vi "Method Memory.vi"(8 "error in":errorcluster, 11 "Method Name":string) -> (0 "error out":errorcluster, 1 "method exists?":bool, 3 "Method Out":T1)   [LabVIEW 2012]
uses:
  Method.ctl
  ReadWrite.ctl
  Which method type.ctl
panel:
  out "method":i32
  out "version":i32
  out "Version List":i32[](array[numeric])
  in  "Method Failure":T1={"Title"="Method Failure", "About"="5", "Input Parameters"=[], "AutoCAD drawings"=[], "Stock file names"=[], "Publish files"=[], "Display images"=[]}
  out "Method Array (method, version)":T1[][](array[typedef])
  out "Method List":string[](array[string])
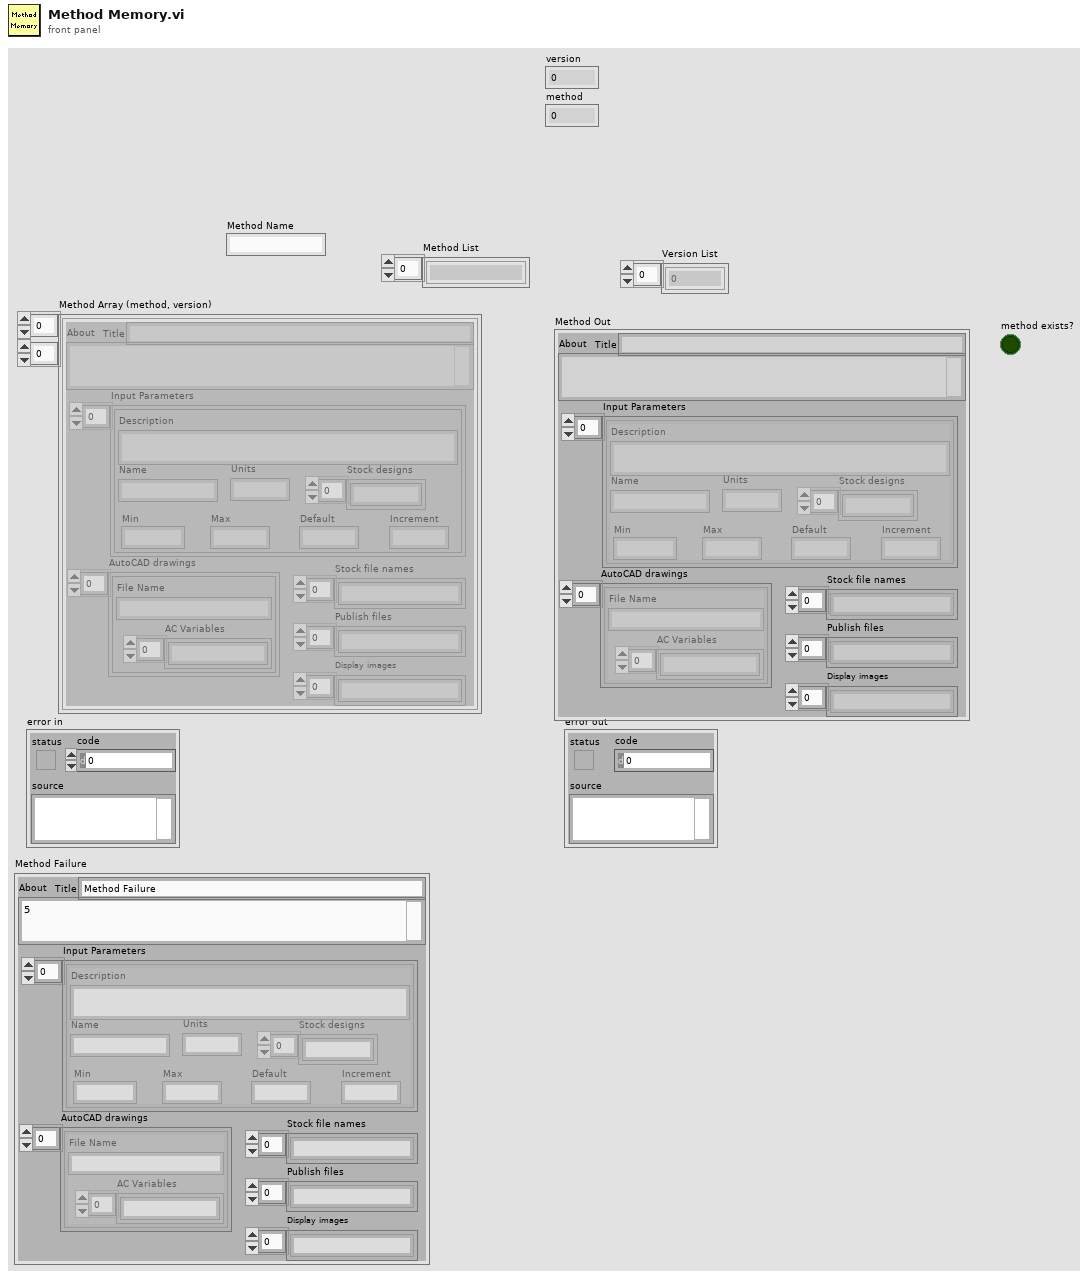
[diagram p1: front panel]
types:
  T1 = typedef "Method.ctl" = cluster{"Title":string, "About":string, "Input Parameters":cluster{"Description":string, "Name":string, "Min":string, "Max":string, "Default":string, "Units":string, "Increment":string, "Stock designs":string[]}[], "AutoCAD drawings":cluster{"File Name":string, "AC Variables":string[]}[], "Stock file names":string[], "Publish files":string[], "Display images":string[]}
  T2 = typedef "ReadWrite.ctl" = enum16{"Read", "Write"}
  T3 = typedef "Which method type.ctl" = enum16{"Master Method", "Method"}
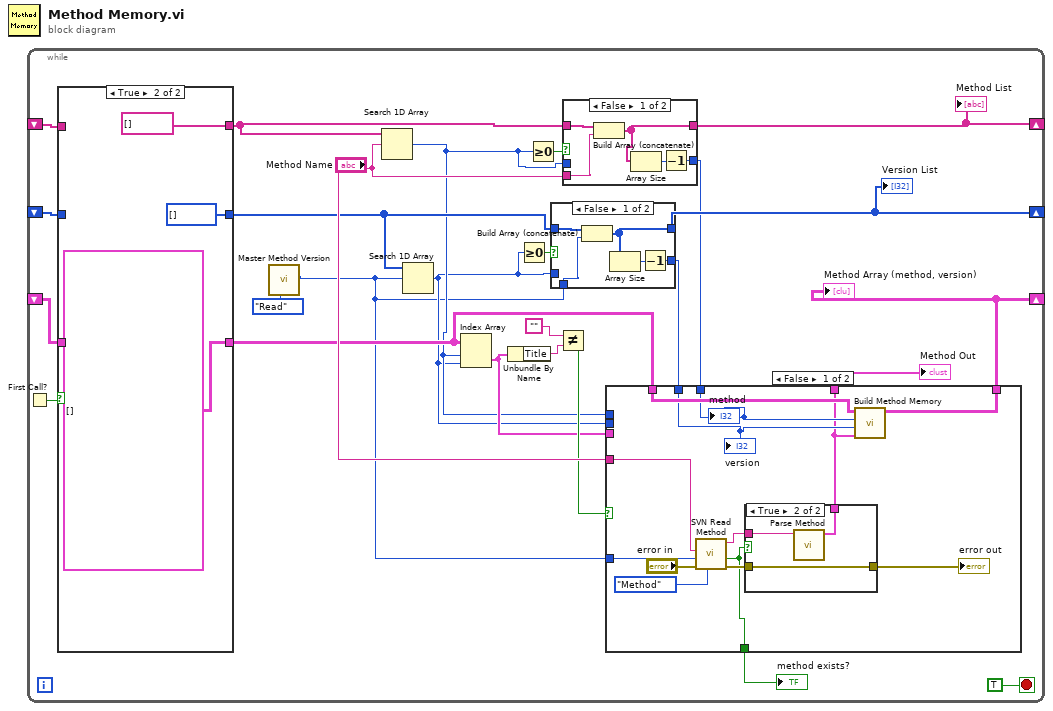
[diagram p0: block diagram]
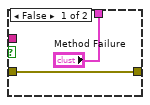
[diagram p4: hidden frame]
diagram:
  n1 = while {
    shift-right: [w23] -> _
    shift-left: _ -> [w16]
    shift-right: [w8] -> _
    shift-left: _ -> [w18]
    shift-right: [w9] -> _
    shift-left: _ -> [w11]
    stop <- TRUE stop-if-true
    n2 = First Call?() -> (First Call?: T/F=w19:bool)
    n3 = case shown="True" w19 {
      tunnel: [w36 T1[][] [] ("Method Array (method, version)")] -> w7
      tunnel: w18 -> [w36 _]
      tunnel: [w35 string[] [] ("Method List")] -> w17
      tunnel: w16 -> [w35 _]
      tunnel: [w34 i32[] []] -> w10
      tunnel: w11 -> [w34 _]
      frame False {
      }
      frame True {
      }
    }
    n4 = call "Master Method Version.vi"("Config"=ReadWrite."Read") -> ("Current Master Method Version"=w1:i32)  [unwired: 7 in, 3 out]
    n5 = Search 1D Array(1D array=w17, element="Method Name") -> (index of element=w4:i32)  [unwired: 1 in]
    n6 = Search 1D Array(1D array=w10, element=w1) -> (index of element=w3:i32)  [unwired: 1 in]
    n7 = Index Array(array=w7, index (row)=w4, index (col)=w3) -> (element=w14:T1)
    n8 = Unbundle By Name(w14) -> ("Title"=w22:string)
    n9 = Greater Or Equal To 0?(x=w3) -> (x >= 0?=w12:bool)
    n10 = Greater Or Equal To 0?(x=w4) -> (x >= 0?=w25:bool)
    n11 = case shown="False" w12 {
      tunnel: w10 -> [w31 w33]
      tunnel: [w29 w33] -> w9
      tunnel: w1 -> [w30 _]
      tunnel: [w28 w32] -> w5
      tunnel: w3 -> [_ w32]
      frame False {
        n12 = Build Array (concatenate)(w31, w30) -> (w29:i32[])
        n13 = Array Size(array=w29) -> (size(s)=w27:i32)
        n14 = Decrement(x=w27) -> (x-1=w28:i32)
      }
      frame True {
      }
    }
    "Version List" <- w9
    n15 = Not Equal?(x="", y=w22) -> (x != y?=w15:bool)
    n16 = case shown="False" w25 {
      tunnel: w17 -> [w65 w67]
      tunnel: [w63 w67] -> w23
      tunnel: "Method Name" -> [w64 _]
      tunnel: [w61 w66] -> w6
      tunnel: w4 -> [_ w66]
      frame False {
        n17 = Build Array (concatenate)(w65, w64) -> (w63:string[])
        n18 = Array Size(array=w63) -> (size(s)=w62:i32)
        n19 = Decrement(x=w62) -> (x-1=w61:i32)
      }
      frame True {
      }
    }
    "Method List" <- w23
    n20 = case shown="False" w15 {
      selector: w15 -> [_ w59]
      tunnel: "Method Name" -> [w47 _]
      tunnel: w1 -> [w46 _]
      tunnel: [w40 w60] -> w20
      tunnel: w14 -> [_ w60]
      tunnel: [w45 w59] -> w13
      tunnel: w3 -> [_ _]
      tunnel: [w44 w58] -> w8
      tunnel: w4 -> [_ _]
      tunnel: w7 -> [w43 w58]
      tunnel: w6 -> [w42 _]
      tunnel: w5 -> [w41 _]
      frame False {
        n21 = call "SVN Read Method.vi"("Which Method Type"=Which_method_type."Method", "error in (no error)"="error in", "Method version"=w46, "Method Name"=w47) -> ("error out"=w48:errorcluster, "Valid method"=w45:bool, "Method text"=w50:string)  [unwired: 5 in]
        n22 = case shown="True" w45 {
          tunnel: [w54 w57] -> w52
          tunnel: w50 -> [_ w56]
          tunnel: w48 -> [w54 w57]
          tunnel: ["Method Failure" w55] -> w40
          frame False {
          }
          frame True {
            n23 = call "Parse Method.vi"("Method text"=w56) -> ("Method Cluster"=w55:T1)  [unwired: 10 in]
          }
        }
        "error out" <- w52
        n24 = call "Build Method Memory.vi"("Method in"=w40, "version"=w41, "method"=w42, "Method Array in"=w43) -> ("Method Array out"=w44:T1[][])  [unwired: 7 in]
        "version" <- w41
        "method" <- w42
      }
      frame True {
      }
    }
    "Method Array (method, version)" <- w8
    "Method Out" <- w20
    "method exists?" <- w13
  }
